vi "InitDMA.vi"(8 "error in (no error)":errorcluster, 11 "FpgaRef5782 in":refnum<class "FpgaRefx410.lvclass">) -> (0 "error out":errorcluster, 3 "FpgaRef5782 out":refnum<class "FpgaRefx410.lvclass">)   [LabVIEW 2025, in "FpgaRefx410.lvclass"]
uses:
  FpgaRefx410.lvclass
  FpgaRefx410.lvclass/FpgaRefx410.ctl
  <vilib>/rvi/interface/common/niFpgaWaitOnOcc.vi
  <vilib>/Utility/error.llb/Error Cluster From Error Code.vi
  <vilib>/rvi/interface/nirviMethod/nirviMethod.xnode
  x410 FPGA ref.ctl
  <vilib>/rvi/errors/niLvFpgaMergeErrorWithErrorCode.vi
  <vilib>/FPGAPlugInAG/Dynamic/niLvFpga_StartFifo_Dynamic.vi
  <vilib>/FPGAPlugInAG/Dynamic/niLvFpga_ConfigureFifo_Dynamic.vi
  <vilib>/FPGAPlugInAG/Dynamic/niLvFpga_ReadFifo_Dynamic.vi
panel:
  out "Actual Depth":u32
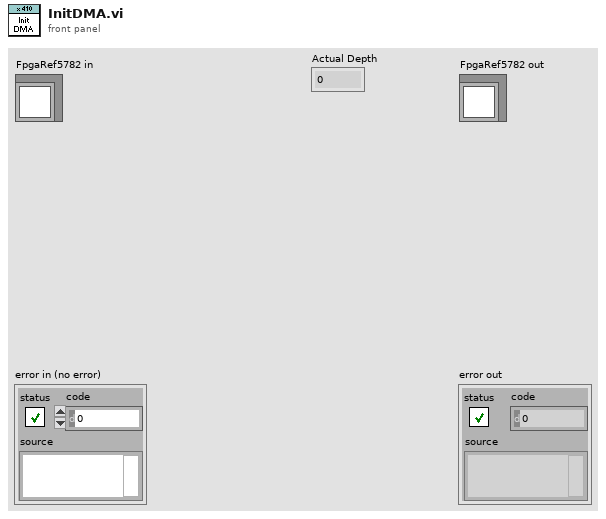
[diagram p1: front panel]
types:
  T1 = typedef "x410 FPGA ref.ctl" = refnum<k20>
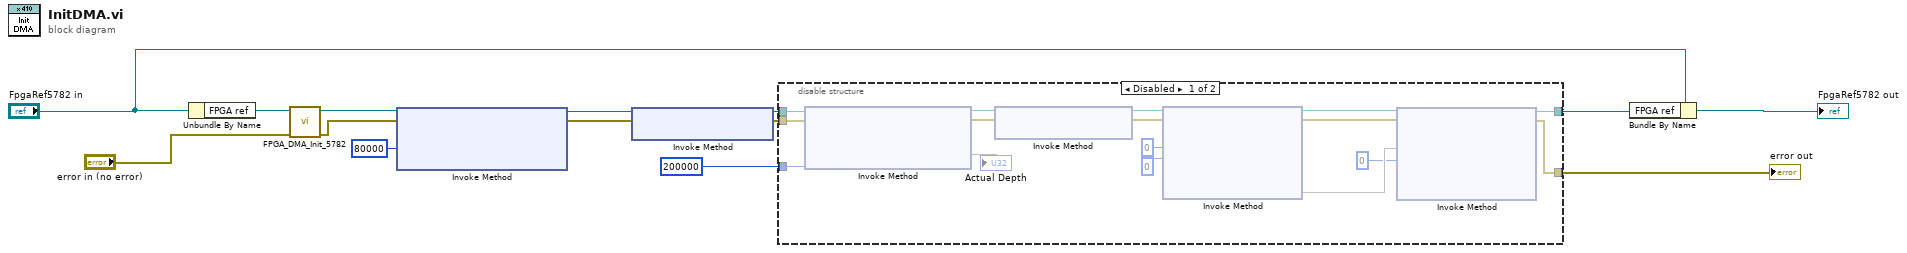
[diagram p0: block diagram]
diagram:
  n1 = Unbundle By Name("FpgaRef5782 in") -> ("FPGA ref"=w14:T1)
  n2 = call "FPGA_DMA_Init_5782.vi"("error in (no error)"="error in (no error)", "FPGA VI Reference"=w14) -> ("error out"=w6:errorcluster, "FPGA VI Out"=w8:T1)  [unwired: 7 in, 1 out]
  n3 = xnode "Invoke Method"("FPGA VI Reference In"=w8, "error in"=w6, "Requested Depth"=u32 80000 ("Depth")) -> ("FPGA VI Reference Out"=w7:T1, "error out"=w9:errorcluster)  [unwired: 1 out]
  n4 = xnode "Invoke Method"("FPGA VI Reference In"=w7, "error in"=w9) -> ("FPGA VI Reference Out"=w5:T1, "error out"=w4:errorcluster)
  n5 = disable-structure shown="Disabled" {
    disable-tunnel: w5 -> [w30 w32]
    disable-tunnel: w4 -> [w29 w31]
    disable-tunnel: u32 200000 ("Depth") -> [w28 _]
    disable-tunnel: [w17 w32] -> w2
    disable-tunnel: [w16 w31] -> w1
    frame Disabled {
      n6 = xnode "Invoke Method"("FPGA VI Reference In"=w30, "error in"=w29, "Requested Depth"=w28) -> ("FPGA VI Reference Out"=w27:T1, "error out"=w26:errorcluster, "Actual Depth"=→"Actual Depth")
      n7 = xnode "Invoke Method"("FPGA VI Reference In"=w27, "error in"=w26) -> ("FPGA VI Reference Out"=w19:T1, "error out"=w18:errorcluster)
      n8 = xnode "Invoke Method"("FPGA VI Reference In"=w19, "error in"=w18, "Number of Elements"=u32 0, "Timeout (ms)"=0) -> ("FPGA VI Reference Out"=w21:T1, "error out"=w20:errorcluster, "Elements Remaining"=w23)  [unwired: 1 out]
      n9 = xnode "Invoke Method"("FPGA VI Reference In"=w21, "error in"=w20, "Number of Elements"=w23, "Timeout (ms)"=0) -> ("FPGA VI Reference Out"=w17:T1, "error out"=w16:errorcluster)  [unwired: 2 out]
    }
    frame Enabled {
    }
  }
  "error out" <- w1
  n10 = Bundle By Name(cluster="FpgaRef5782 in", "FPGA ref"=w2) -> (→"FpgaRef5782 out":refnum<class "FpgaRefx410.lvclass">)
